vi "WriteStr.vi"(7 "路径":string="data\\data.ini", 8 "error in":errorcluster caption="错误输入（无错误）", 9 "value":string caption="Value", 10 "key":string caption="Key", 11 "Section":string) -> (0 "error out":errorcluster caption="错误输出", 3 "ConfigPath":string)   [LabVIEW 2013]
uses:
  <vilib>/Utility/config.llb/Write Key (String).vi
  <vilib>/Utility/config.llb/NI_LVConfig.lvlib
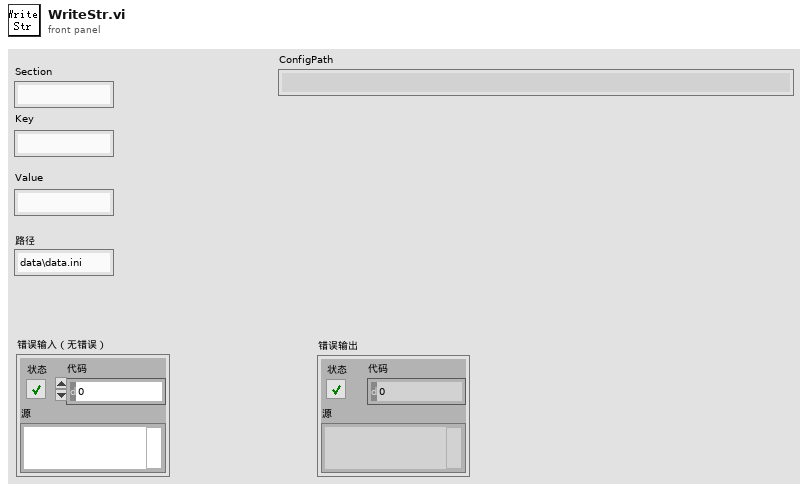
[diagram p1: front panel]
types:
  T1 = enum32{"invalid app kind", "Development System", "Run Time System", "Student Edition", "Embedded LabVIEW", "Evaluation", "Custom"}
  T2 = typedef "NI_LVConfig.lvlib/Config Data RefNum.ctl" = refnum<k1>
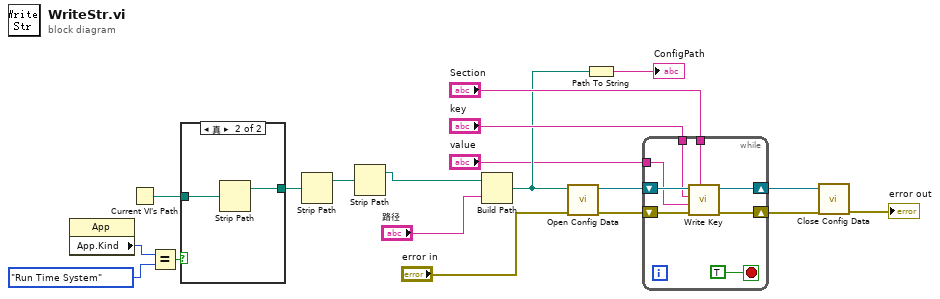
[diagram p0: block diagram]
diagram:
  n1 = property class="App"() -> ("App.Kind"=w19:T1)  [unwired: 2 in, 2 out]
  n2 = Current VI's Path() -> (path=w16:path)
  n3 = Equal?(x=w19, y=T1."Run Time System" ("应用程序:类别")) -> (x = y?=w17:bool)
  n4 = case shown="真" w17 {
    tunnel: w16 -> [w20 w22]
    tunnel: [w20 w21] -> w15
    frame False {
    }
    frame True {
      n5 = Strip Path(path=w22) -> (stripped path=w21:path)  [unwired: 1 out]
    }
  }
  n6 = Strip Path(path=w15) -> (stripped path=w10:path)  [unwired: 1 out]
  n7 = Strip Path(path=w10) -> (stripped path=w1:path)  [unwired: 1 out]
  n8 = Build Path(base path=w1, name or relative path="路径") -> (appended path=w7:path)
  n9 = call <vilib>:"Open Config Data.vi"("error in (no error)"="error in", "configuration file path"=w7) -> ("error out"=w11:errorcluster, "refnum"=w14:T2)  [unwired: 7 in, 1 out]
  n10 = Path To String(path=w7) -> (string=→"ConfigPath":string)
  n11 = while {
    tunnel: "Section" -> [w29]
    tunnel: "key" -> [w28]
    tunnel: "value" -> [w24]
    shift-right: [w26] -> w4
    shift-left: w14 -> [w30]
    shift-right: [w25] -> w3
    shift-left: w11 -> [w27]
    stop <- TRUE stop-if-true
    n12 = call-poly <vilib>:"Write Key.vi"("section"=w29, "error in (no error)"=w27, "value"=w24, "key"=w28, "refnum"=w30) -> ("error out"=w25:errorcluster, "refnum out"=w26:T2)  [unwired: 4 in, 1 out]
  }
  n13 = call <vilib>:"Close Config Data.vi"("error in (no error)"=w3, "refnum"=w4) -> ("error out"=→"error out":errorcluster)  [unwired: 8 in, 1 out]
